vi "Read Configuration with Known Module.vi"() -> ()   [LabVIEW 2019]
uses:
  Types/Module Channel Settings.ctl
  <vilib>/addons/VeriStand Custom Device Scripting APIs/Scan Engine/Modules/Mode Classes/Controls/counter driven output channel settings.ctl
  <vilib>/addons/VeriStand Custom Device Scripting APIs/Scan Engine/Modules/Channel Classes/Counter Driven Output Channel/Counter Driven State.ctl
  <vilib>/addons/VeriStand Custom Device Scripting APIs/Scan Engine/Modules/Mode Classes/Controls/pwm channel settings.ctl
  <vilib>/addons/VeriStand Custom Device Scripting APIs/Scan Engine/Modules/Channel Classes/PWM Output Channel/Frequency.ctl
  <vilib>/addons/VeriStand Custom Device Scripting APIs/Scan Engine/Modules/NI 9474/NI 9474.lvclass
  C:/Program Files (x86)/National Instruments/LabVIEW 2019/vi.lib/addons/VeriStand Custom Device Scripting APIs/Scan Engine/Modules/Module/Module.lvclass
  f6bbfe02-b953-4ef2-a52c-5a4fac125821.vi
  a1ceeb16-d950-4579-9989-ec83f905a63a.vi
  <vilib>/addons/VeriStand Custom Device Scripting APIs/Scan Engine/Scan Engine Dependencies.llb/Set Error.vi
  <vilib>/Utility/error.llb/Clear Errors.vi
  <vilib>/addons/VeriStand Custom Device Scripting APIs/Scan Engine/Utility/Convert Slot Configuration to 9212.vi
  <vilib>/addons/VeriStand Custom Device Scripting APIs/Scan Engine/Utility/Convert Slot Configuration to 9213.vi
  <vilib>/addons/VeriStand Custom Device Scripting APIs/Scan Engine/Modules.lvlibp/SD Module/SD Module.lvclass
  C:/Program Files (x86)/National Instruments/LabVIEW 2019/vi.lib/addons/VeriStand Custom Device Scripting APIs/Scan Engine/Modules.lvlibp/RSI Module/RSI Module.lvclass
  <vilib>/addons/VeriStand Custom Device Scripting APIs/Scan Engine/Modules/NI 9212/NI 9212.lvclass
  <vilib>/addons/VeriStand Custom Device Scripting APIs/Scan Engine/Modules/NI 9213/NI 9213.lvclass
  <vilib>/addons/VeriStand Custom Device Scripting APIs/Scan Engine/Modules/NI 9224/NI 9224.lvclass
  <vilib>/addons/VeriStand Custom Device Scripting APIs/Scan Engine/Modules/NI 9228/NI 9228.lvclass
  <vilib>/addons/VeriStand Custom Device Scripting APIs/Scan Engine/Modules.lvlibp/RSI Module/Read Module Page Property.vi
  <vilib>/addons/VeriStand Custom Device Scripting APIs/Scan Engine/Modules.lvlibp/RSI Module/Read Model.vi
  <vilib>/addons/VeriStand Custom Device Scripting APIs/Scan Engine/Utility/Convert Module Model to Module Class.vi
  <vilib>/addons/VeriStand Custom Device Scripting APIs/Scan Engine/Modules.lvlibp/SD Module/Read DIO mode.vi
  <vilib>/addons/VeriStand Custom Device Scripting APIs/Scan Engine/Modules.lvlibp/RSI Module/Read Channels.vi
  <vilib>/addons/VeriStand Custom Device Scripting APIs/Scan Engine/Utility/Convert to DI Module.vi
  <vilib>/addons/VeriStand Custom Device Scripting APIs/Scan Engine/Utility/Convert to DO Module.vi
  <vilib>/addons/VeriStand Custom Device Scripting APIs/Scan Engine/Utility/Convert to CI PWM Module.vi
  <vilib>/addons/VeriStand Custom Device Scripting APIs/Scan Engine/Utility/Convert to CDO Module.vi
  <vilib>/addons/VeriStand Custom Device Scripting APIs/Scan Engine/Utility/Convert to PWM Module.vi
  <vilib>/addons/VeriStand Custom Device Scripting APIs/Scan Engine/Scan Engine Dependencies.llb/Error Strings.vi
  <vilib>/addons/VeriStand Custom Device Scripting APIs/Scan Engine/Utility/Get Channel Names and Default Values for Slot.vi
  <vilib>/addons/VeriStand Custom Device Scripting APIs/Scan Engine/Modules/NI 9212/Create NI 9212.vi
  <vilib>/addons/VeriStand Custom Device Scripting APIs/Scan Engine/Modules/NI 9213/Create NI 9213.vi
  <vilib>/addons/VeriStand Custom Device Scripting APIs/Scan Engine/Utility/Convert to AI Module.vi
  <vilib>/addons/VeriStand Custom Device Scripting APIs/Scan Engine/Utility/Convert to AI Vrms Module.vi
  <vilib>/addons/VeriStand Custom Device Scripting APIs/Scan Engine/Utility/Convert to AI Arms Module.vi
  <vilib>/addons/VeriStand Custom Device Scripting APIs/Scan Engine/Utility/Convert to DIO Module.vi
  <vilib>/addons/VeriStand Custom Device Scripting APIs/Scan Engine/Modules/NI 9474/Read NI 9474 - PWM Output.vi
  <vilib>/addons/VeriStand Custom Device Scripting APIs/Scan Engine/Modules/NI 9474/Read NI 9474 - Counter Driven Output.vi
  <vilib>/addons/VeriStand Custom Device Scripting APIs/Scan Engine/Modules/Module/Module.lvclass
  <vilib>/addons/VeriStand Custom Device Scripting APIs/Scan Engine/Modules.lvlibp/9212/9212.lvclass
  <vilib>/addons/VeriStand Custom Device Scripting APIs/Scan Engine/Modules.lvlibp/9213/9213.lvclass
  <vilib>/addons/VeriStand Custom Device Scripting APIs/Scan Engine/Modules.lvlibp/9224/9224.lvclass
  SubVIs/Scan Engine Example Support.lvlib
  <vilib>/addons/VeriStand Custom Device Scripting APIs/Scan Engine/Scan Engine Scripting.lvlib
  <vilib>/addons/VeriStand Custom Device Scripting APIs/Scan Engine/Modules/Channel Classes/PWM Output Channel/PWM Output Channel.lvclass
  <vilib>/addons/VeriStand Custom Device Scripting APIs/Scan Engine/Modules/Channel Classes/Counter Driven Output Channel/Counter Driven Output Channel.lvclass
panel:
  out "Channel Settings":T1[](array[typedef])
  # "Overview: Demonstrates using the Scan Engine and EtherCAT scripting API to read a configuration from a system definition file that contains a Scan Engine Custom Device.\nThis example assumes it is known what module types the configuration file contains.\n\nInstructions:\nRun the VI."
  # "Slot Properties"
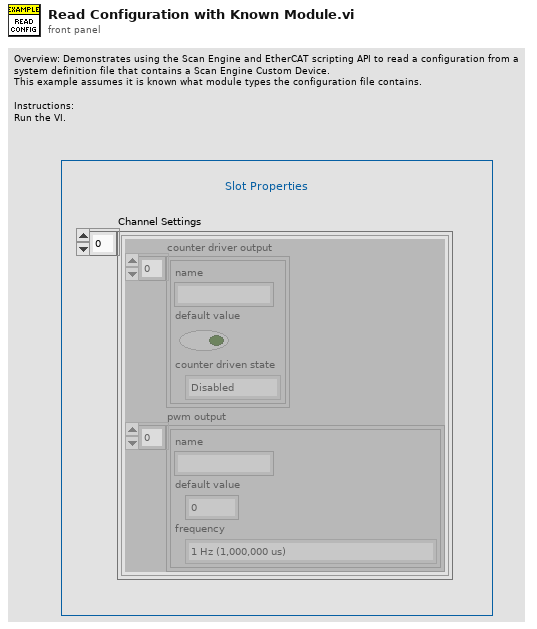
[diagram p1: front panel]
types:
  T1 = typedef "Module Channel Settings.ctl" = cluster{"counter driver output":T2[], "pwm output":T4[]}
  T2 = typedef "Scan Engine Scripting.lvlib/counter driven output channel settings.ctl" = cluster{"name":string, "default value":bool, "counter driven state":T3}
  T3 = typedef "Scan Engine Scripting.lvlib/Counter Driven Output Channel.lvclass/Counter Driven State.ctl" = enum16{"Disabled", "Enabled"}
  T4 = typedef "Scan Engine Scripting.lvlib/pwm channel settings.ctl" = cluster{"name":string, "default value":dbl, "frequency":T5}
  T5 = typedef "Scan Engine Scripting.lvlib/PWM Output Channel.lvclass/Frequency.ctl" = enum16{"1 Hz (1,000,000 us)", "50 Hz (20,000 us)", "250 Hz (4,000 us)", "500 Hz (2,000 us)", "1 kHz (1,000 us)", "5 kHz (200 us)", "10 kHz (100 us)", "20 kHz (50 us)"}
  T6 = typedef "Custom Device API.lvlib/Custom Device Item Ref.ctl" = u64
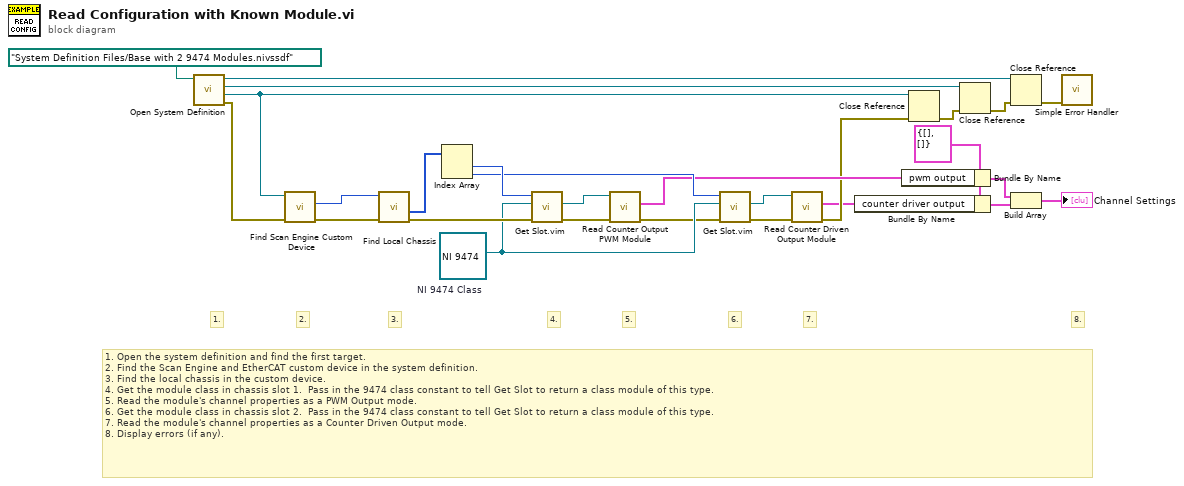
[diagram p0: block diagram]
diagram:
  w13 = refnum<class "NI 9474.lvclass"> refnum  # NI 9474 Class
  w6 = T1 {"counter driver output"=[], "pwm output"=[]} ("Cluster")
  # "7."
  # "6."
  # "5."
  # "4."
  # "3."
  # "2."
  # "8."
  # "1."
  # "1. Open the system definition and find the first target.\n2. Find the Scan Engine and EtherCAT custom device in the system definition.\n3. Find the local chassis in the custom device.\n4. Get the module class in chassis slot 1.  Pass in the 9474 class constant to tell Get Slot to return a class module of this type.\n5. Read the module's channel properties as a PWM Output mode.\n6. Get the module class in chassis slot 2.  Pass in the 9474 class constant to tell Get Slot to return a class module of this type.\n7. Read the module's channel properties as a Counter Driven Output mode.\n8. Display errors (if any)."
  n1 = call "Open System Definition.vi"("System Definition File"=path "System Definition Files/Base with 2 9474 Modules.nivssdf" ("Input System Definition File")) -> ("error out"=w19:errorcluster, "Target Refnum"=w18:refnum<k24>, "Root Refnum"=w21:refnum<k24>, "System Definition Refnum"=w22:refnum<k24>)  [unwired: 7 in]
  n2 = call <vilib>:"Find Scan Engine Custom Device.vi"("error in"=w19, "target in"=w18) -> ("error out"=w20:errorcluster, "scan engine custom device ref"=w23:T6)  [unwired: 6 in, 2 out]
  n3 = call <vilib>:"Find Local Chassis.vi"("error in"=w20, "scan engine custom device ref in"=w23) -> ("error out"=w17:errorcluster, "slots refs"=w16:T6[])  [unwired: 4 in, 4 out]
  n4 = Index Array(array=w16) -> (element #1=w15:T6, element #2=w14:T6)  [unwired: 2 in]
  n5 = call "Get Slot.vim"("error in"=w17, "module type"=w13, "slot ref in"=w15) -> ("error out"=w9:errorcluster, "module"=w2:refnum<class "NI 9474.lvclass">)  [unwired: 5 in, 2 out]
  n6 = call-poly <vilib>:"Read Counter Output PWM Module.vi"("error in"=w9, "NI 9474 in"=w2) -> ("error out"=w8:errorcluster, "channel settings"=w11:T4[])  [unwired: 7 in, 1 out]
  n7 = call "Get Slot.vim"("error in"=w8, "module type"=w13, "slot ref in"=w14) -> ("error out"=w7:errorcluster, "module"=w12:refnum<class "NI 9474.lvclass">)  [unwired: 5 in, 2 out]
  n8 = call-poly <vilib>:"Read Counter Driven Output Module.vi"("error in"=w7, "NI 9474 in"=w12) -> ("error out"=w4:errorcluster, "channel settings"=w1:T2[])  [unwired: 6 in, 2 out]
  n9 = Bundle By Name(cluster=w6, "counter driver output"=w1) -> (w5:T1)
  n10 = Bundle By Name(cluster=w6, "pwm output"=w11) -> (w3:T1)
  n11 = Close Reference(reference=w18, error in (no error)=w4) -> (error out=w26:errorcluster)
  n12 = Close Reference(reference=w21, error in (no error)=w26) -> (error out=w27:errorcluster)
  n13 = Close Reference(reference=w22, error in (no error)=w27) -> (error out=w25:errorcluster)
  n14 = Build Array(w3, w5) -> (→"Channel Settings":T1[])
  n15 = call <vilib>:"Simple Error Handler.vi"("error in (no error)"=w25) -> ()  [unwired: 1 in, 8 out]
